vi "ATF-Pump-Create DO Waveform.vi"(8 "dt(sec)":dbl=2000.0, 9 "Size":i32, 10 "DO Channel Names":string[](array[string]), 11 "DO Values In":bool[](array[boolean])) -> (2 "DO Digital Waveform":digitalwaveform[](array[waveform]), 3 "DO Waveform":waveform(dbl)[](array[waveform]))   [LabVIEW 2022 SP3]
uses:
  <vilib>/Waveform/DTblOps.llb/DTbl Boolean Array to Digital.vi
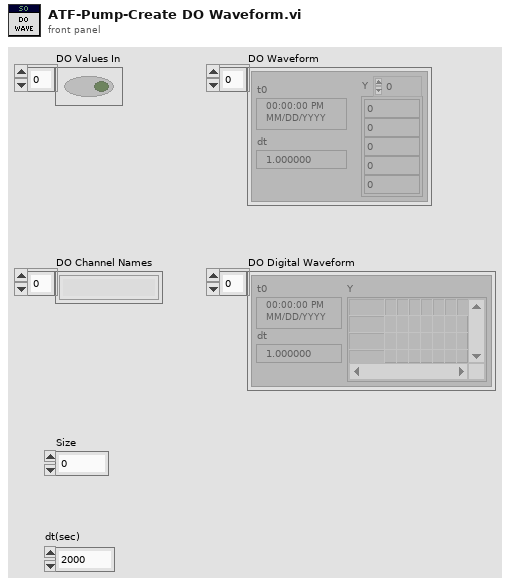
[diagram p1: front panel]
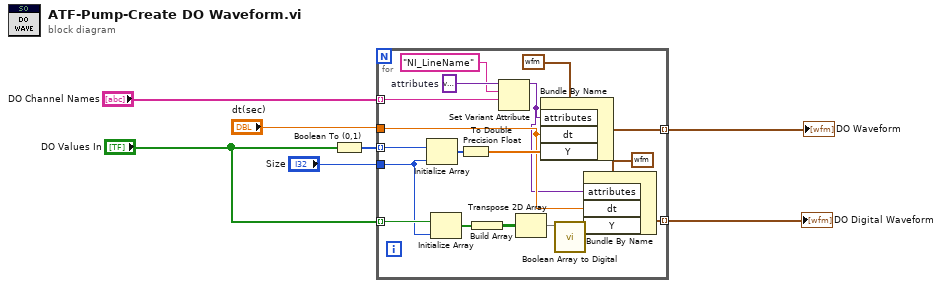
[diagram p0: block diagram]
diagram:
  n1 = Boolean To (0,1)(Boolean="DO Values In") -> (0, 1=w2:i16[])
  n2 = for {
    tunnel: w2 -> [w24] mode=indexing
    tunnel: [w25] -> w4 mode=indexing
    tunnel: "Size" -> [w20]
    tunnel: "DO Values In" -> [w21] mode=indexing
    tunnel: [w15] -> w5 mode=indexing
    tunnel: "DO Channel Names" -> [w12] mode=indexing
    tunnel: "dt(sec)" -> [w9]
    w13 = variant  # attributes
    n3 = Initialize Array(w24, w20) -> (w23:i16[])
    n4 = Initialize Array(w21, w20) -> (w19:bool[])
    n5 = To Double Precision Float(number=w23) -> (double precision float=w22:dbl[])
    n6 = Build Array(w19) -> (w18:bool[][])
    n7 = Set Variant Attribute(Variant=w13, name="NI_LineName", value=w12) -> (Variant out=w8:variant)  [unwired: 1 in, 2 out]
    n8 = Transpose 2D Array(2D array=w18) -> (transposed array=w14:bool[][])
    n9 = Bundle By Name(cluster=waveform(dbl) {"t0"=timestamp(0 s since 1904-01-01), "dt"=1.0, "Y"=[]} ("waveform"), "attributes"=w8, "dt"=w9, "Y"=w22) -> (w25:waveform(dbl))
    n10 = call-poly <vilib>:"Boolean Array to Digital.vi"("boolean array"=w14) -> ("digital data"=w16:digitaldata)  [unwired: 9 in, 1 out]
    n11 = Bundle By Name(cluster=digitalwaveform {"t0"=timestamp(0 s since 1904-01-01), "dt"=0.0, "Y"={"transitions"=[], "data"=[]}, "error"={"status"=FALSE, "code"=37421928, "source"=""}} ("Waveform"), "attributes"=w8, "dt"=w9, "Y"=w16) -> (w15:digitalwaveform)
  }
  "DO Digital Waveform" <- w5
  "DO Waveform" <- w4
